vi "init_coor.vi"(11 "芯片角点坐标":T1) -> (3 "x+y":dbl[](array[numeric]))   [LabVIEW 2013]
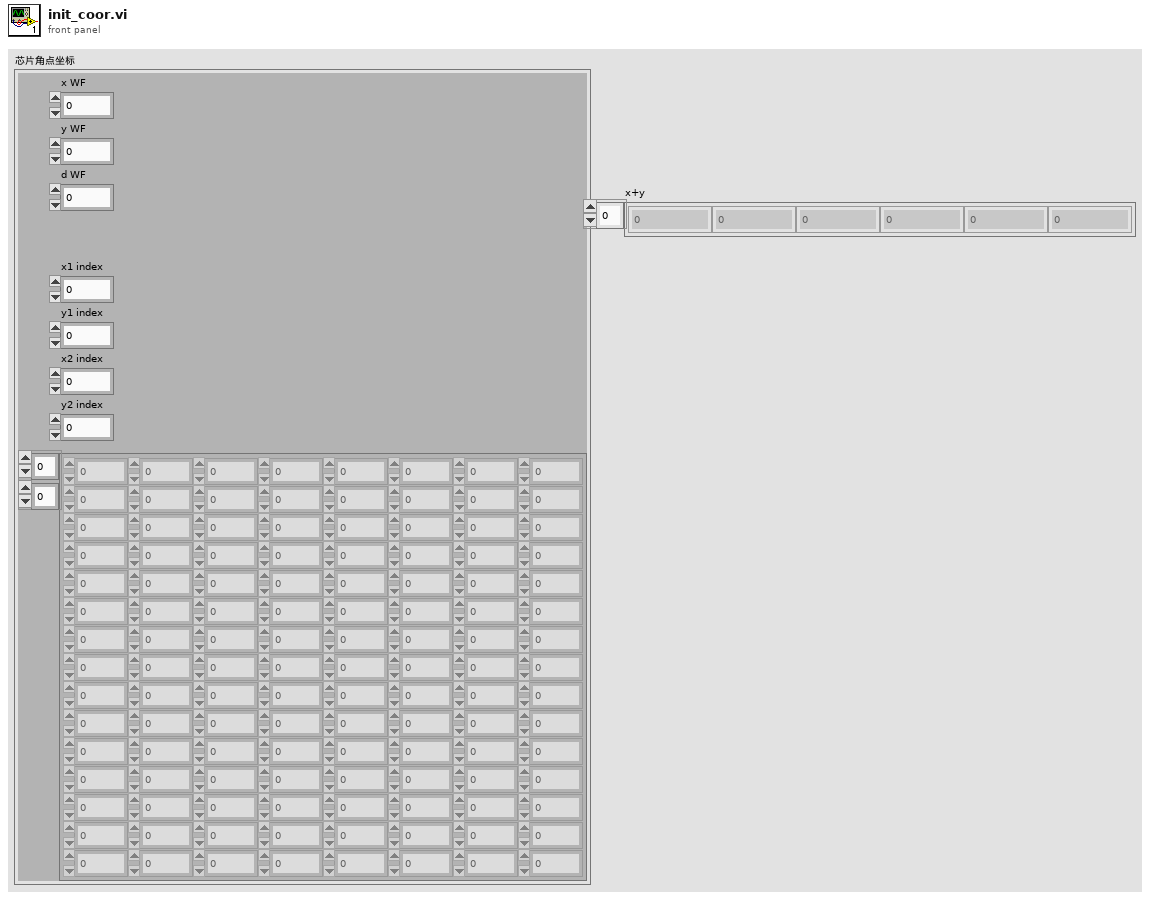
[diagram p1: front panel]
types:
  T1 = cluster{"x WF":dbl, "y WF":dbl, "d WF":dbl, "x1 index":i32, "y1 index":i32, "x2 index":i32, "y2 index":i32, dbl[][]}
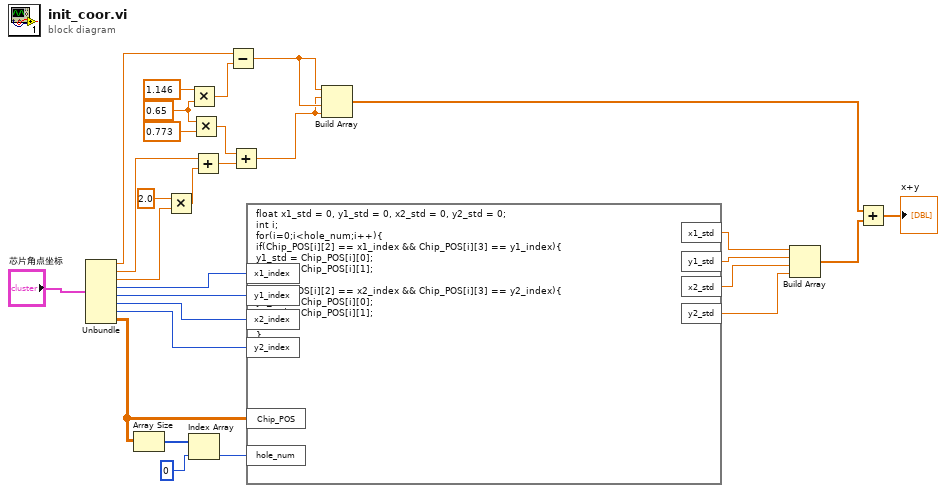
[diagram p0: block diagram]
diagram:
  w16 = 0.65 ("y")
  n1 = Unbundle("芯片角点坐标") -> ("x WF"=w20:dbl, "y WF"=w19:dbl, "d WF"=w18:dbl, "x1 index"=w24:i32, "y1 index"=w23:i32, "x2 index"=w22:i32, "y2 index"=w21:i32, w26:dbl[][])
  n2 = Array Size(array=w26) -> (size(s)=w27:i32[])
  n3 = Multiply(x=2.0, y=w18) -> (x*y=w13:dbl)
  n4 = Multiply(x=1.146, y=w16) -> (x*y=w12:dbl)
  n5 = Index Array(array=w27, index=0 ("索引")) -> (element=w25:i32)
  n6 = Multiply(x=w16, y=0.773) -> (x*y=w10:dbl)
  n7 = Add(x=w19, y=w13) -> (x+y=w11:dbl)
  n8 = Subtract(x=w20, y=w12) -> (x-y=w9:dbl)
  n9 = Add(x=w10, y=w11) -> (x+y=w8:dbl)
  n10 = formula code="float x1_std = 0, y1_std = 0, x2_std = 0, y2_std = 0;\nint i;\nfor(i=0;i<hole_num;i++){\nif(Chip_POS[i][2] == x1_index && Chip_POS[i][3] == y1_index){\ny1_std = Chip_POS[i][0]; \nx1_std = Chip_POS[i][1];\n}\nif(Chip_POS[i][2] == x2_index && Chip_POS[i][3] == y2_index){\ny2_std = Chip_POS[i][0]; \nx2_std = Chip_POS[i][1];\n}\n}"("Chip_POS"=w26, "hole_num"=w25, "x1_index"=w24, "y1_index"=w23, "x2_index"=w22, "y2_index"=w21) -> ("y1_std"=w6:dbl, "x2_std"=w5:dbl, "y2_std"=w4:dbl, "x1_std"=w7:dbl)
  n11 = Build Array(w9, w8, w9, w8) -> (w3:dbl[])
  n12 = Build Array(w7, w6, w5, w4) -> (w2:dbl[])
  n13 = Add(x=w3, y=w2) -> (x+y=→"x+y":dbl[])
